vi "Initialize Session.vi"(8 "error in":errorcluster, 10 "shared resources":refnum<class "Shared Resources.lvclass">, 11 "Tx Execution Unit Implementation in":refnum<class "Tx Execution Unit.lvclass">) -> (0 "error out":errorcluster, 3 "Tx Execution Unit Implementation out":refnum<class "Tx Execution Unit.lvclass">)   [LabVIEW 2020, in "afdx_custom_device Engine.lvlib" / "Implementation.lvlib" / "Tx Execution Unit.lvclass"]
uses:
  Tx Execution Unit.lvclass
  AIM LabVIEW src/src/AIM664LV.lvlib
  AIM LabVIEW src/src/_polimorphicInstances/session/Fdx Create Session (Tx-Generic).vi
  AIM LabVIEW src/src/_controls/queue_header_generic.ctl
  Interfaces/Shared Resources/Shared Resources.lvclass
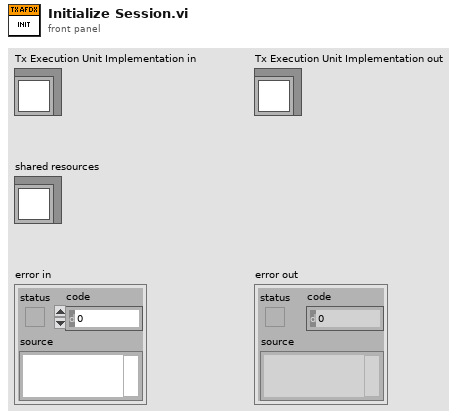
[diagram p1: front panel]
types:
  T1 = typedef "AIM664LV.lvlib/queue_header_generic.ctl" = cluster{"InterFrameGap":u32, "PacketGroupWaitTime":u32, "PayloadBufferMode":u8, "PayloadGenerationMode":u8, "PreambleCount":u8, "Skew":u32, "NetSelect":u8, "FrameStartMode":u8, "PhysErrorInjection":u32, "SequenceNumberInit":u16, "SequenceNumberOffset":u16}
  T2 = typedef "channel_settings_tx.ctl" = cluster{"Rx Board":dbl, "Rx Port":dbl}
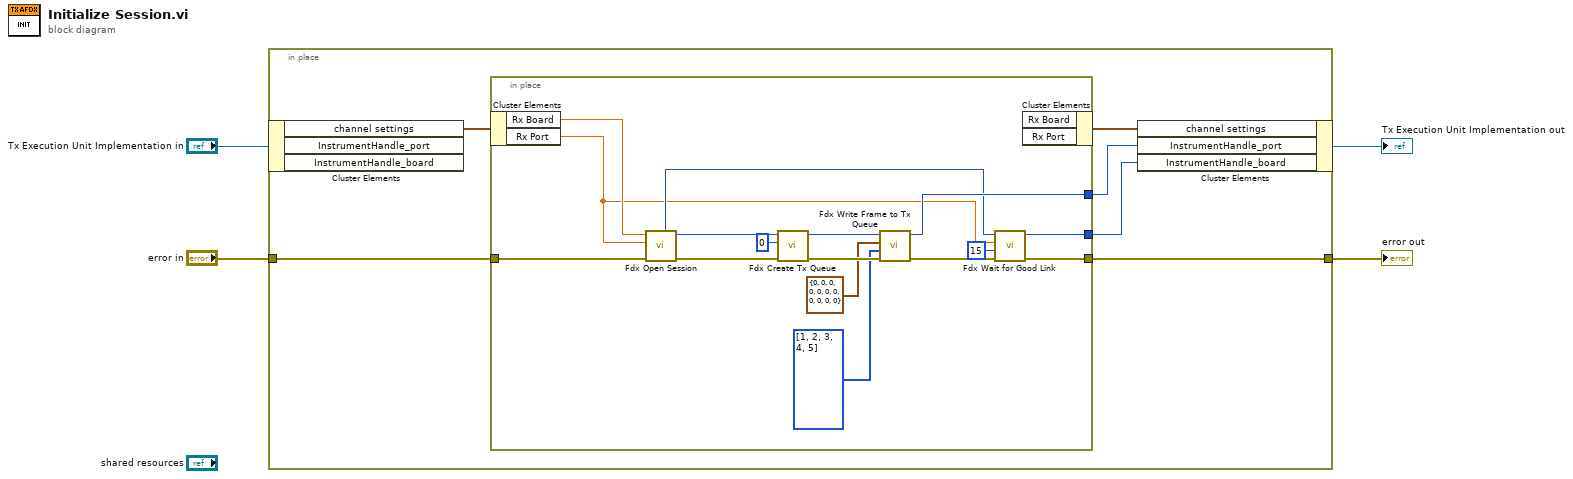
[diagram p0: block diagram]
diagram:
  n1 = in-place {
    in-place-border: "error in" -> [w10]
    in-place-border: [w9] -> w2
    n2 = in-place-cluster #1("Tx Execution Unit Implementation in") -> ("channel settings"=w8:T2)  [unwired: 2 out]
    n3 = in-place {
      in-place-border: w10 -> [w19]
      in-place-border: [w23] -> w9
      in-place-border: [w22] -> w6
      in-place-border: [w20] -> w5
      n4 = in-place-cluster #2(w8) -> ("Rx Board"=w18:dbl, "Rx Port"=w14:dbl)
      n5 = call-poly "Fdx Open Session.vi"("error in (no error)"=w19, "port"=w14, "board"=w18) -> ("error out"=w17:errorcluster, "port handle out"=w16:u32, "InstrumentHandle_board out"=w15:u32)  [unwired: 4 in, 2 out]
      n6 = call "Fdx Create Tx Queue.vi"("error in (no error)"=w17, "QueueSizeIn"=u32 0, "InstrumentHandle_port in"=w16) -> ("error out"=w26:errorcluster, "InstrumentHandle_port out"=w24:u32)  [unwired: 6 in, 1 out]
      n7 = call "Fdx Write Frame to Tx Queue.vi"("error in (no error)"=w26, "Frame in"=u8[] [1, 2, 3, 4, 5], "HeaderInfo"=T1 {"InterFrameGap"=0, "PacketGroupWaitTime"=0, "PayloadBufferMode"=0, "PayloadGenerationMode"=0, "PreambleCount"=0, "Skew"=0, "NetSelect"=0, "FrameStartMode"=0, "PhysErrorInjection"=0, "SequenceNumberInit"=0, "SequenceNumberOffset"=0}, "InstrumentHandle_port in"=w24) -> ("error out"=w25:errorcluster, "InstrumentHandle_port out"=w20:u32)  [unwired: 6 in]
      n8 = call "Fdx Wait for Good Link.vi"("error in"=w25, "timeout s(10)"=u32 15, "port id"=w14, "InstrumentHandle_board in"=w15) -> ("error out"=w23:errorcluster, "InstrumentHandle_board out"=w22:u32)  [unwired: 4 in, 2 out]
      n9 = in-place-cluster #2() -> (w7:T2)  [unwired: 2 in]
    }
    n10 = in-place-cluster #1("channel settings"=w7, "InstrumentHandle_port"=w5, "InstrumentHandle_board"=w6) -> (→"Tx Execution Unit Implementation out":refnum<class "Tx Execution Unit.lvclass">)
  }
  "error out" <- w2
